vi "Test1_1b_ASIC.vi"(0 "Instrument VISA in":T1={"AWG VISA"="generadorpulsos", "Oscilloscope  VISA "="Oscilloscope", "Integration Board IP"="172.16.7.43", "connection ID"=refnum, "report out"=refnum, "report file path"=path "C:/Documents and Settings/CTA_LAB01/Desktop/L0_Asic/L0 Asic Test Data"}, 1 "threshold":i32[][](array[numeric]), 2 "Serial Number":string, 5 "quantity":i32=3, 7 "Cycles Burst":i32=10000, 11 "error in":errorcluster={"status"=FALSE, "code"=0, "source"="VISA Write in Test2_3a_ASIC_fast.vi->test_sum_ASIC.vi"}, 12 "channel array":i32[](array[numeric])=[0, 1, 2, 3, 4, 5, 6], 13 "Voltages comprobation":dbl[](array[numeric])=[0.05, 0.1, 0.2, 0.5, 0.8, 0.5, 0.6, 0.7, 0.8, 1.0]) -> (4 "Instrument VISA out":T1, 15 "error out":errorcluster)   [LabVIEW 2009]
uses:
  <vilib>/Utility/NIReport.llb/NI_report.lvclass
  <vilib>/Utility/NIReport.llb/HTML/NI_HTML.lvclass
  <instrlib>/Agilent 81150/Agilent 81150.lvlib
  L0_Asic/L0 Asic Test Folder v9/C/Program Files/National Instruments/LabVIEW 2012/instr.lib/Agilent 8000 Series/Agilent 8000 Series.lvlib
panel:
  out "read buffer 4":string="V amptd(f2),1.074E+00,0,1.056E+00,1.087E+00,1.0690E+00,5.5E-03,9.4E+01,+ width(f2),2.90015E-09,0,2.90015E-09,2.95960E-09,2.925838E-09,1.2702E-11,9.4E+01,V amptd(1),5.5E-02,0,4.8E-02,6.7E-02,5.55E-02,3.5E-03,9.4E+01,+ width(f1),9.99999E+37,5,9.99999E+37,9.99999E+37,9.99999E+37,9.99999E+37,9.99999E+37,Time(f1-f2),6.26722E-09,0,6.20145E-09,6.35270E-09,6.264189E-09,3.2805E-11,9.4E+01\n"
  out "report file path":path=path "C:/Documents and Settings/CTA_LAB01/Desktop/L0_Asic/L0 Asic Test Data"
  out "Array":i32[](array[numeric])=[2, 3, 5]
  out "points quantity":dbl=94.0
  out "ouput data array":dbl[](array[numeric])=[0.75, 42.0, 0.0, 63.0, 1.0, 1.069, 0.0055, 2.925838e-09, 1.2702e-11, 0.0555, 0.0035, 9.99999e+37, 9.99999e+37, 6.264189e-09, 3.2805e-11, 94.0]
  out "read buffer 3":string="V amptd(f2),1.074E+00,0,1.056E+00,1.087E+00,1.0690E+00,5.5E-03,9.4E+01,+ width(f2),2.90015E-09,0,2.90015E-09,2.95960E-09,2.925838E-09,1.2702E-11,9.4E+01,V amptd(1),5.5E-02,0,4.8E-02,6.7E-02,5.55E-02,3.5E-03,9.4E+01,+ width(f1),9.99999E+37,5,9.99999E+37,9.99999E+37,9.99999E+37,9.99999E+37,9.99999E+37,Time(f1-f2),6.26722E-09,0,6.20145E-09,6.35270E-09,6.264189E-09,3.2805E-11,9.4E+01\n"
  in  "Voltage":dbl[](array[numeric])=[0.05, 0.1, 0.2, 0.5, 0.8]
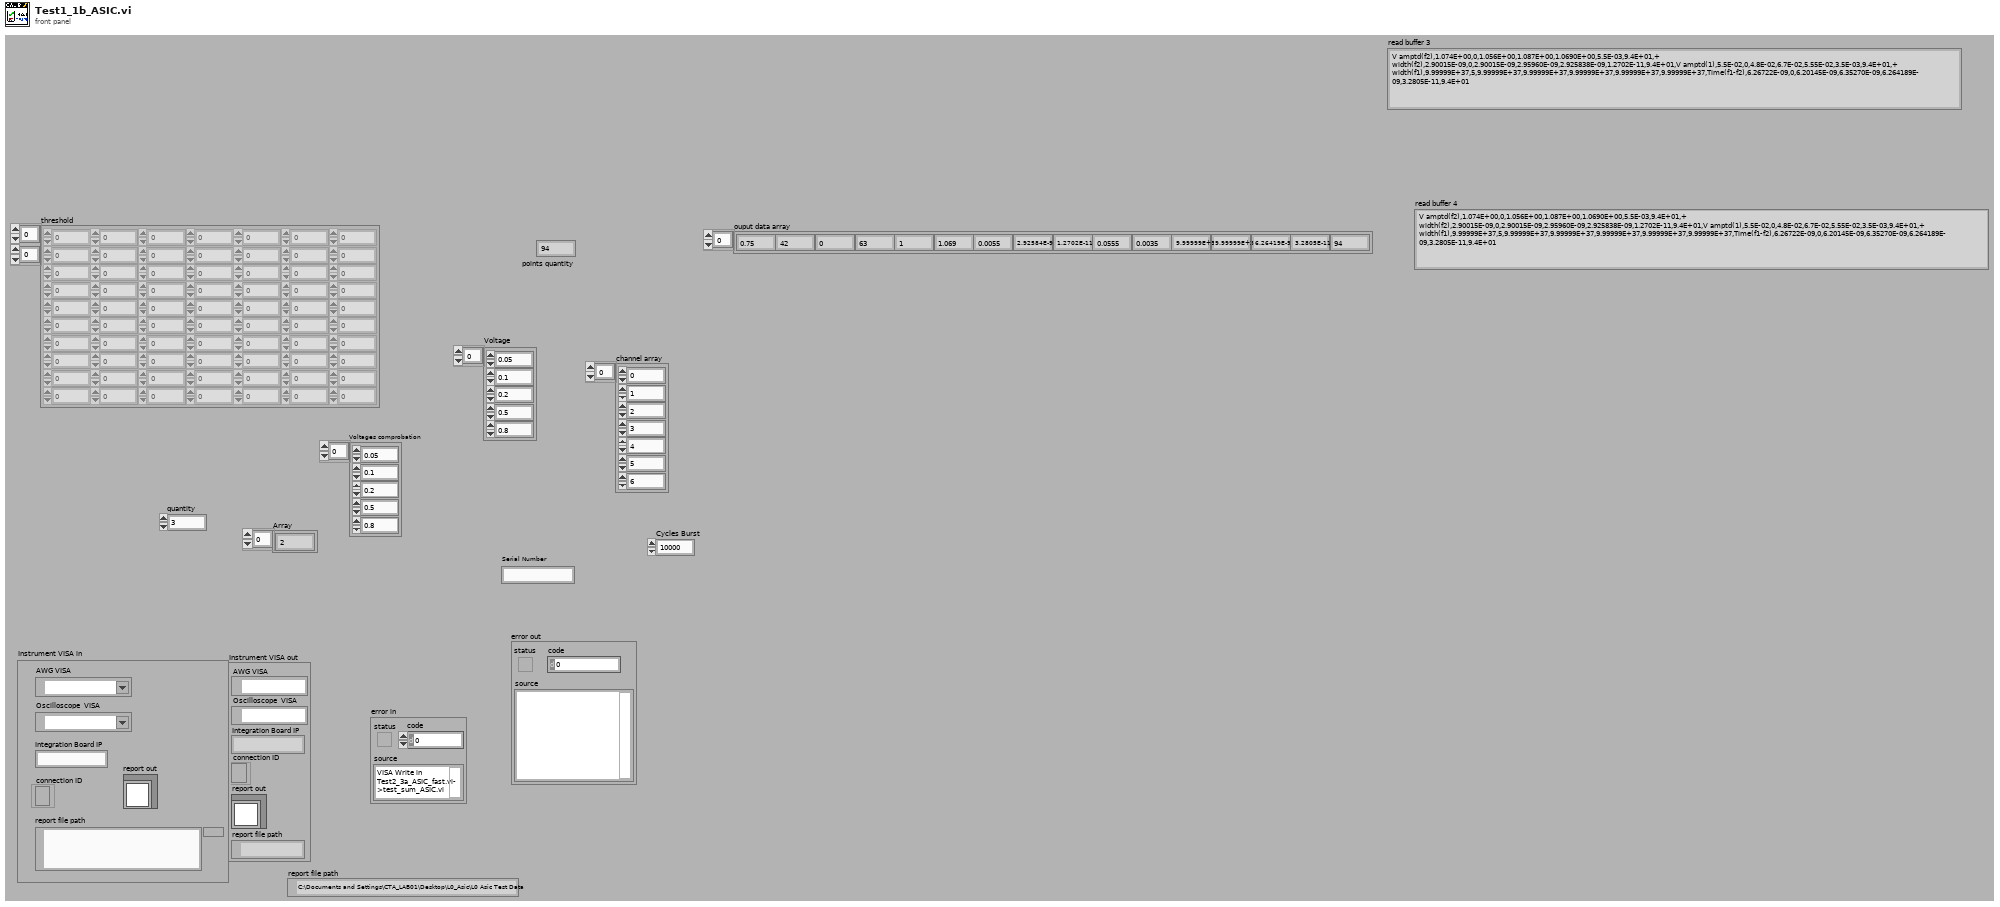
[diagram p1: front panel]
types:
  T1 = cluster{"AWG VISA":refnum<visa-resource-name>, "Oscilloscope  VISA ":refnum<visa-resource-name>, "Integration Board IP":string, "connection ID":refnum<k5>, "report out":refnum<class "NI_report.lvclass">, "report file path":path}
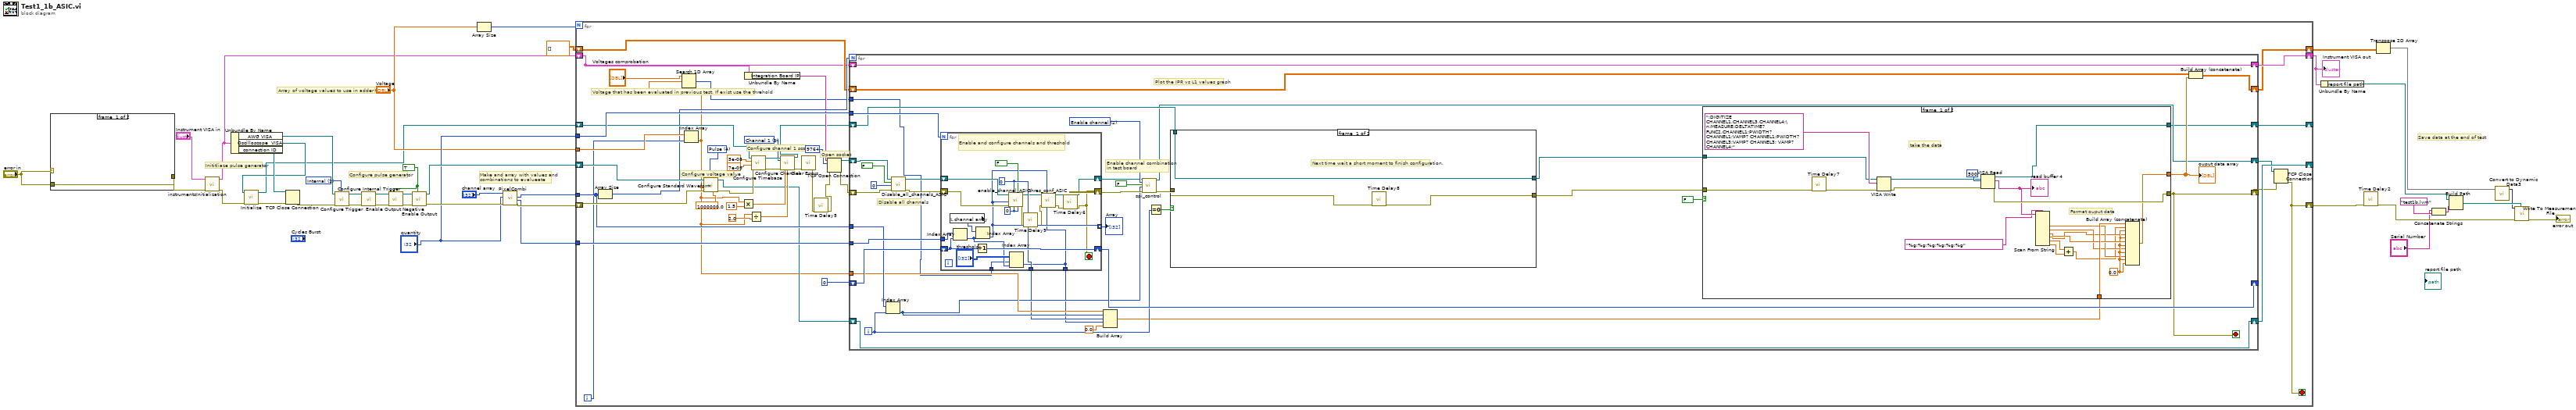
[diagram p0: block diagram]
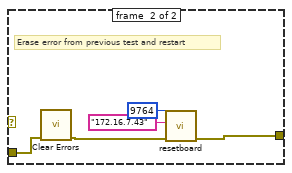
[diagram p2: hidden frame]
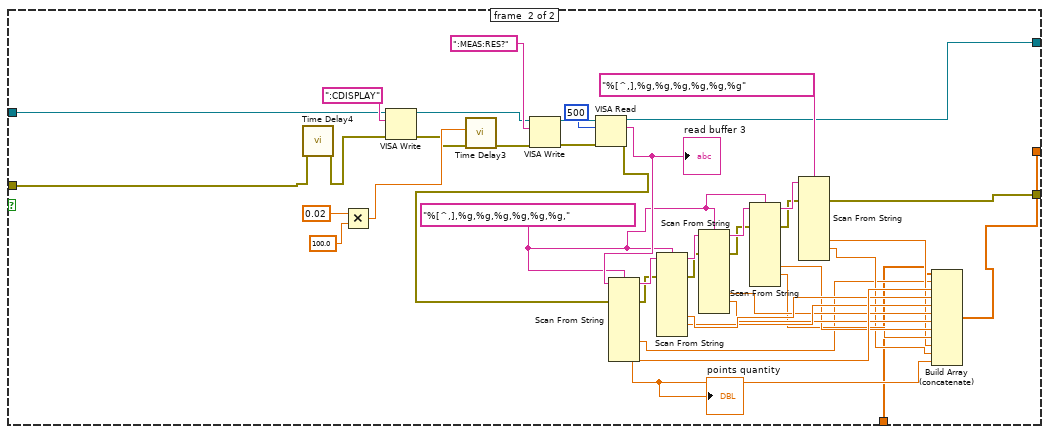
[diagram p3: hidden frame]
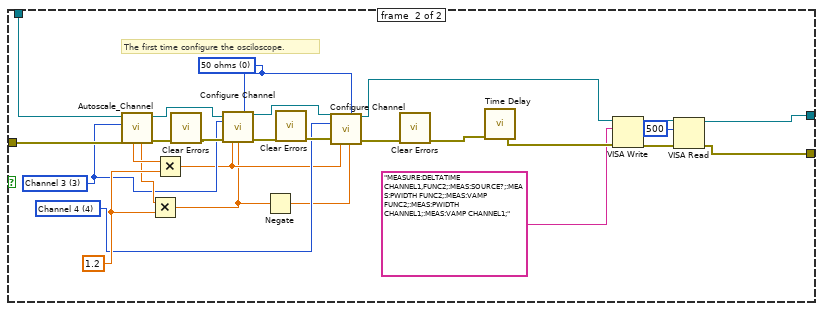
[diagram p4: hidden frame]
diagram:
  w22 = u16 1 items=["Immediate", "Internal", "External", "Software Trigger Function"] ("Trigger Source (0: Immediate)")
  w9 = TRUE ("Enable Output (T: Enable)")
  # "Save data at the end of test"
  # "Array of voltage values to use in adder test"
  # "Make and array with values and \ncombinations to evalueate"
  # "Configure pulse generator"
  # "Inititliaze pulse generator"
  n1 = case shown="No Error" "error in" {
    tunnel: "error in" -> [w42 w44]
    tunnel: [w42 w47] -> w18
    frame #0 {
    }
    frame #1 {
      # "Erase error from previous test and restart"
      n2 = call <vilib>:"Clear Errors.vi"("error in (no error)"=w44) -> ("error out"=w43:errorcluster)  [unwired: 6 in]
      n3 = call "resetboard.vi"("error in (no error)"=w43, "address"="172.16.7.43", "remote port or service name"=u16 9764) -> ("error out"=w47:errorcluster)  [unwired: 7 in, 1 out]
    }
  }
  n4 = call "instrumentsInitialization.vi"("error in"=w18, "Instrument VISA in"="Instrument VISA in") -> ("error out"=w7:errorcluster, "Instrument VISA out"=w15:T1)  [unwired: 8 in]
  n5 = Unbundle By Name(w15) -> ("AWG VISA"=w25:refnum<visa-resource-name>, "Oscilloscope  VISA"=w5:refnum<visa-resource-name>, "connection ID"=w17:refnum<k5>)
  n6 = call "Initialize.vi"("error in (no error)"=w7, "VISA resource name"=w5) -> ("error out"=w6:errorcluster, "VISA resource name out"=w4:refnum<visa-resource-name>)  [unwired: 8 in]
  n7 = TCP Close Connection(connection ID=w17, error in (no error)=w6) -> (error out=w16:errorcluster)  [unwired: 1 in, 1 out]
  n8 = call <instrlib>:"Configure Trigger.vi"("Trigger Source (0: Immediate)"=w22, "error in (no error)"=w16, "VISA resource name"=w25) -> ("error out"=w23:errorcluster, "VISA resource name out"=w24:refnum<visa-resource-name>)  [unwired: 7 in]
  n9 = call <instrlib>:"Configure Internal Trigger.vi"("error in (no error)"=w23, "VISA resource name"=w24) -> ("error out"=w11:errorcluster, "VISA resource name out"=w12:refnum<visa-resource-name>)  [unwired: 8 in]
  n10 = call <instrlib>:"Enable Output Negative.vi"("Enable Output (T: Enable)"=w9, "error in (no error)"=w11, "VISA resource name"=w12) -> ("error out"=w10:errorcluster, "VISA resource name out"=w13:refnum<visa-resource-name>)  [unwired: 7 in]
  n11 = call <instrlib>:"Enable Output.vi"("Enable Output (T: Enable)"=w9, "error in (no error)"=w10, "VISA resource name"=w13) -> ("error out"=w41:errorcluster, "VISA resource name out"=w39:refnum<visa-resource-name>)  [unwired: 7 in]
  n12 = Array Size(array="Voltage") -> (size(s)=w32:i32)
  n13 = call "PixelCombi.vi"("error in"=w41, "quantity"="quantity", "array"="channel array") -> ("error out"=w40:errorcluster, "Channels"=w38:i32[], "Combination Array"=w37:i16[])  [unwired: 6 in]
  n14 = for {
    N: w32 -> [_]
    tunnel: w38 -> [w88]
    tunnel: w37 -> [w87]
    shift-right: [w76] -> w26
    shift-left: w40 -> [w90]
    tunnel: "Voltage" -> [w86]
    tunnel: "quantity" -> [w84]
    shift-right: [w80] -> w14
    shift-left: w15 -> [w51]
    shift-right: [w79] -> w8
    shift-left: dbl[][] [] -> [w81]
    shift-right: [w77] -> _
    shift-left: w39 -> [w89]
    shift-right: [w78] -> _
    shift-left: w4 -> [w83]
    i -> [w85]
    stop <- w76 stop-if-true
    w66 = 1 items=["Channel 1"=1, "Channel 2"=2, "Channel 3"=3, "Channel 4"=4] ("Channel (1: Channel 1)")
    w75 = u16 4 items=["Sine", "Square", "Ramp Up", "Ramp Down", "Pulse", "Noise", "DC"] ("Waveform (0: Sine)")
    # "Open socket"
    # "Configure channel 1 scope"
    # "Configure voltage value"
    # "Voltage that has been evaluated in previous test. If exist use the threhold"
    n15 = Array Size(array=w87) -> (size(s)=w82:i32)
    n16 = Index Array(array=w86, index=w85) -> (element=w50:dbl)
    n17 = Search 1D Array(1D array="Voltages comprobation", element=w50) -> (index of element=w48:i32)  [unwired: 1 in]
    n18 = call <instrlib>:"Configure Standard Waveform.vi"("Frequency (1000.0 Hz)"=1000000.0, "Waveform (0: Sine)"=w75, "error in (no error)"=w90, "Amplitude (1.0 Vpp)"=w50, "VISA resource name"=w89) -> ("error out"=w72:errorcluster, "VISA resource name out"=w54:refnum<visa-resource-name>)  [unwired: 5 in]
    n19 = Multiply(x=w50, y=1.5) -> (x*y=w65:dbl)
    n20 = Unbundle By Name(w51) -> ("Integration Board IP"=w62:string)
    n21 = Divide(x=w50, y=2.0) -> (x/y=w59:dbl)
    n22 = call "Configure Timebase.vi"("error in (no error)"=w72, "Position (0.0 s)"=7e-09, "Timebase (0.005 s)"=5e-08, "VISA resource name"=w83) -> ("error out"=w71:errorcluster, "VISA resource name out"=w69:refnum<visa-resource-name>)  [unwired: 6 in]
    n23 = call "Configure Channel.vi"("VISA resource name"=w69, "Channel (1: Channel 1)"=w66, "error in (no error)"=w71, "Vertical Range (2.0 V)"=w65, "Vertical Offset (0.0 V)"=w59) -> ("VISA resource name out"=w58:refnum<visa-resource-name>, "error out"=w70:errorcluster)  [unwired: 9 in]
    n24 = call <vilib>:"Clear Errors.vi"("error in (no error)"=w70) -> ("error out"=w53:errorcluster)  [unwired: 6 in]
    n25 = call "Time Delay5"("error in (no error)"=w53) -> ("error out"=w52:errorcluster)  [unwired: 10 in]
    n26 = TCP Open Connection(address=w62, remote port or service name=u16 9764, error in (no error)=w52) -> (connection ID=w55:refnum<k5>, error out=w63:errorcluster)  [unwired: 2 in]
    n27 = for {
      N: w82 -> [_]
      tunnel: w87 -> [w125]
      tunnel: w88 -> [w126]
      shift-right: [w127] -> _
      shift-left: i16 0 ("element") -> [w128]
      shift-right: [w106] -> w57
      shift-left: w63 -> [w118]
      tunnel: w84 -> [w124]
      shift-right: [w119] -> w79
      shift-left: w81 -> [w120]
      shift-right: [w107] -> w56
      shift-left: w55 -> [w105]
      tunnel: w50 -> [w103]
      shift-right: [w99] -> w78
      shift-left: w58 -> [w112]
      shift-right: [w98] -> w77
      shift-left: w54 -> [w98]
      shift-right: [w93] -> w80
      shift-left: w51 -> [w93]
      tunnel: w48 -> [w91]
      i -> [w110]
      stop <- w106 stop-if-true
      w117 = u16 2 items=["Attenuation", "Clipping", "Enable channel", "Delay line", "ASIC"] ("Device")
      # "Enable channel combination \nin test board"
      # "Disable all channels"
      # "Plot the IPR vs L1 values graph"
      n28 = Index Array(array=w125, index=w110) -> (element=w102:i16)
      n29 = call "Disable_all_channels_ASIC.vi"("error in"=w118, "id_in"=0 ("Data"), "Clip_en_b"=FALSE, "connection ID"=w105) -> ("error out"=w122:errorcluster, "connection ID out"=w121:refnum<k5>)  [unwired: 5 in, 1 out]
      n30 = for {
        N: w124 -> [_]
        shift-right: [w239] -> w127
        shift-left: w128 -> [w240]
        tunnel: w126 -> [w238]
        shift-right: [w227] -> w115
        shift-left: w122 -> [w236]
        shift-right: [w230] -> w114
        shift-left: w121 -> [w235]
        tunnel: [w229] -> w104 mode=indexing
        tunnel: [w234] -> w101
        tunnel: [w228] -> w94
        tunnel: w91 -> [w223]
        stop <- w227 stop-if-true
        w232 = u32 0 ("Ib_clipVb")
        w234 = u32 0 ("Att gain")
        # "Enable and configure channels and threshold"
        n31 = local read "channel array"() -> (w237:i32[])
        n32 = Index Array(array=w238, index=w240) -> (element=w224:i32)
        n33 = Increment(x=w240) -> (x+1=w239:i16)
        n34 = Index Array(array=w237, index=w224) -> (element=w229:i32)
        n35 = call "enable_channel_ASIC.vi"("Clip_sel_b"=w232, "maj/sum"=FALSE, "Ib_clipVb"=w232, "Att gain"=w234, "error in"=w236, "Channel"=w229, "connection ID"=w235) -> ("error out"=w221:errorcluster, "connection ID out"=w231:refnum<k5>)  [unwired: 2 in, 1 out]
        n36 = Index Array(array="threshold", index (row)=w223, index (col)=w224) -> (element=w228:i32)
        n37 = call "Time Delay9"("error in (no error)"=w221) -> ("error out"=w222:errorcluster)  [unwired: 10 in]
        n38 = call "thres_conf_ASIC.vi"("threshold"=w228, "Ring"=w229, "error out 3"=w222, "connection ID"=w231) -> ("error out 2"=w226:errorcluster, "connection ID out"=w230:refnum<k5>)  [unwired: 4 in, 2 out]
        n39 = call "Time Delay6"("error in (no error)"=w226) -> ("error out"=w227:errorcluster)  [unwired: 10 in]
      }
      "Array" <- w104
      n40 = Build Array(w103, w102, w101, w94, 0.0 ("element")) -> (w100:dbl[])
      n41 = call "spi_control.vi"("connection ID"=w114, "Device"=w117, "Read/#write"=FALSE, "Data"=w102, "error out 3"=w115) -> ("connection ID out"=w107:refnum<k5>, "error out 2"=w113:errorcluster)  [unwired: 7 in, 6 out]
      n42 = Equal To 0?(x=w110) -> (x = 0?=w111:bool)
      n43 = case shown="True" w111 {
        tunnel: [w191 w200] -> w96
        tunnel: w113 -> [w192 w206]
        tunnel: w112 -> [w193 w207]
        tunnel: [w193 w209] -> w109
        frame #0 {
          # "Next time wait a short moment to finish configuration."
          n44 = call "Time Delay8"("error in (no error)"=w192) -> ("error out"=w191:errorcluster)  [unwired: 10 in]
        }
        frame #1 {
          w210 = u32 0 items=["50 ohms", "1 Mohms"] ("Input Impedance (1: 1 Mohms)")
          w198 = 3 items=["Channel 1"=1, "Channel 2"=2, "Channel 3"=3, "Channel 4"=4] ("Channel (1: Channel 1)")
          w197 = 4 items=["Channel 1"=1, "Channel 2"=2, "Channel 3"=3, "Channel 4"=4] ("Channel (1: Channel 1)")
          w203 = 1.2 ("y")
          # "The first time configure the osciloscope."
          n45 = call "Autoscale_Channel.vi"("error in"=w206, "Channel"=w198, "VISA resource name"=w207) -> ("error out"=w217:errorcluster, "VISA resource name out"=w220:refnum<visa-resource-name>, "Offset"=w199:dbl, "VerticalRange"=w214:dbl)  [unwired: 5 in]
          n46 = Multiply(x=w199, y=w203) -> (x*y=w195:dbl)
          n47 = Multiply(x=w214, y=w203) -> (x*y=w196:dbl)
          n48 = call <vilib>:"Clear Errors.vi"("error in (no error)"=w217) -> ("error out"=w218:errorcluster)  [unwired: 6 in]
          n49 = call "Configure Channel.vi"("VISA resource name"=w220, "Input Impedance (1: 1 Mohms)"=w210, "Channel (1: Channel 1)"=w198, "error in (no error)"=w218, "Vertical Range (2.0 V)"=w196, "Vertical Offset (0.0 V)"=w195) -> ("VISA resource name out"=w215:refnum<visa-resource-name>, "error out"=w219:errorcluster)  [unwired: 8 in]
          n50 = Negate(x=w195) -> (-x=w194:dbl)
          n51 = call <vilib>:"Clear Errors.vi"("error in (no error)"=w219) -> ("error out"=w208:errorcluster)  [unwired: 6 in]
          n52 = call "Configure Channel.vi"("VISA resource name"=w215, "Input Impedance (1: 1 Mohms)"=w210, "Channel (1: Channel 1)"=w197, "error in (no error)"=w208, "Vertical Range (2.0 V)"=w196, "Vertical Offset (0.0 V)"=w194) -> ("VISA resource name out"=w204:refnum<visa-resource-name>, "error out"=w216:errorcluster)  [unwired: 8 in]
          n53 = call <vilib>:"Clear Errors.vi"("error in (no error)"=w216) -> ("error out"=w205:errorcluster)  [unwired: 6 in]
          n54 = call "Time Delay"("error in (no error)"=w205) -> ("error out"=w202:errorcluster)  [unwired: 10 in]
          n55 = VISA Write(VISA resource name=w204, write buffer="MEASURE:DELTATIME CHANNEL1,FUNC2;:MEAS:SOURCE?;:MEAS:PWIDTH FUNC2;:MEAS:VAMP FUNC2;:MEAS:PWIDTH CHANNEL1;:MEAS:VAMP CHANNEL1;", error in (no error)=w202) -> (VISA resource name out=w213:refnum<visa-resource-name>, error out=w212:errorcluster)  [unwired: 1 out]
          n56 = VISA Read(VISA resource name=w213, byte count=u32 500, error in (no error)=w212) -> (VISA resource name out=w209:refnum<visa-resource-name>, error out=w200:errorcluster)  [unwired: 2 out]
        }
      }
      n57 = case shown="False" FALSE {
        tunnel: w109 -> [w146 w158]
        tunnel: [w141 w156] -> w108
        tunnel: [w144 w155] -> w106
        tunnel: w100 -> [w142 w153]
        tunnel: [w143 w152] -> w99
        tunnel: w96 -> [w145 w150]
        frame #0 {
          w137 = 0.0 ("output 7")
          # "Format ouput data"
          # "take the data"
          n58 = call "Time Delay7"("error in (no error)"=w145) -> ("error out"=w147:errorcluster)  [unwired: 10 in]
          n59 = VISA Write(VISA resource name=w146, write buffer=":DIGITIZE CHANNEL1,CHANNEL3,CHANNEL4;\n:MEASURE:DELTATIME? FUNC2,CHANNEL1;PWIDTH? CHANNEL1;VAMP? CHANNEL1;PWIDTH? CHANNEL3;VAMP? CHANNEL3; VAMP? CHANNEL4;", error in (no error)=w147) -> (VISA resource name out=w140:refnum<visa-resource-name>, error out=w139:errorcluster)  [unwired: 1 out]
          n60 = VISA Read(VISA resource name=w140, byte count=u32 500, error in (no error)=w139) -> (VISA resource name out=w143:refnum<visa-resource-name>, read buffer=w136:string, error out=w144:errorcluster)  [unwired: 1 out]
          "read buffer 4" <- w136
          n61 = Scan From String(format string="%g;%g;%g;%g;%g;%g", input string=w136) -> (output 1=w134:dbl, output 2=w133:dbl, output 3=w138:dbl, output 4=w132:dbl, output 5=w131:dbl, output 6=w130:dbl)  [unwired: 8 in, 3 out]
          n62 = Add(x=w131, y=w130) -> (x+y=w129:dbl)
          n63 = Build Array (concatenate)(w142, w129, w137, w132, w137, w138, w137, w133, w137, w134, w137, w137) -> (w141:dbl[])
        }
        frame #1 {
          w176 = "%[^,],%g,%g,%g,%g,%g,%g," ("format string")
          n64 = call "Time Delay4"("error in (no error)"=w150) -> ("error out"=w151:errorcluster)  [unwired: 10 in]
          n65 = Multiply(x=0.02, y=100.0) -> (x*y=w183:dbl)
          n66 = VISA Write(VISA resource name=w158, write buffer=":CDISPLAY", error in (no error)=w151) -> (VISA resource name out=w161:refnum<visa-resource-name>, error out=w159:errorcluster)  [unwired: 1 out]
          n67 = call "Time Delay3"("error in (no error)"=w159, "Delay Time (s)"=w183) -> ("error out"=w182:errorcluster)  [unwired: 9 in]
          n68 = VISA Write(VISA resource name=w161, write buffer=":MEAS:RES?", error in (no error)=w182) -> (VISA resource name out=w190:refnum<visa-resource-name>, error out=w189:errorcluster)  [unwired: 1 out]
          n69 = VISA Read(VISA resource name=w190, byte count=u32 500, error in (no error)=w189) -> (VISA resource name out=w152:refnum<visa-resource-name>, read buffer=w186:string, error out=w166:errorcluster)  [unwired: 1 out]
          "read buffer 3" <- w186
          n70 = Scan From String(format string=w176, input string=w186, error in=w166) -> (remaining string=w180:string, error out=w162:errorcluster, output 5=w154:dbl, output 6=w181:dbl, output 7=w167:dbl)  [unwired: 12 in, 1 out]
          "points quantity" <- w167
          n71 = Scan From String(format string=w176, input string=w180, error in=w162) -> (remaining string=w177:string, error out=w163:errorcluster, output 5=w174:dbl, output 6=w173:dbl)  [unwired: 13 in, 1 out]
          n72 = Scan From String(format string=w176, input string=w177, error in=w163) -> (remaining string=w178:string, error out=w164:errorcluster, output 5=w172:dbl, output 6=w171:dbl)  [unwired: 13 in, 1 out]
          n73 = Scan From String(format string=w176, input string=w178, error in=w164) -> (remaining string=w179:string, error out=w165:errorcluster, output 5=w170:dbl, output 6=w169:dbl)  [unwired: 13 in, 1 out]
          n74 = Scan From String(format string="%[^,],%g,%g,%g,%g,%g,%g", input string=w179, error in=w165) -> (error out=w155:errorcluster, output 5=w157:dbl, output 6=w168:dbl)  [unwired: 13 in, 2 out]
          n75 = Build Array (concatenate)(w153, w154, w181, w174, w173, w172, w171, w170, w169, w157, w168, w167) -> (w156:dbl[])
        }
      }
      "ouput data array" <- w108
      n76 = Build Array (concatenate)(w120, w108) -> (w119:dbl[][])
    }
    n77 = TCP Close Connection(connection ID=w56, error in (no error)=w57) -> (error out=w76:errorcluster)  [unwired: 1 in, 1 out]
  }
  "Instrument VISA out" <- w14
  n78 = Unbundle By Name(w14) -> ("report file path"=w35:path)
  n79 = call "Time Delay2"("error in (no error)"=w26) -> ("error out"=w33:errorcluster)  [unwired: 10 in]
  n80 = Transpose 2D Array(2D array=w8) -> (transposed array=w20:dbl[][])
  n81 = Concatenate Strings("Serial Number", "test1b.lvm" ("string")) -> (w3:string)
  n82 = Build Path(base path=w35, name or relative path=w3) -> (appended path=w34:path)
  n83 = call "Convert to Dynamic Data3"("2D Array"=w20) -> ("Dynamic Data Type"=w21:dynamicdata)  [unwired: 3 in]
  n84 = call "Write To Measurement File"("Signals"=w21, "error in (no error)"=w33, "Filename"=w34) -> ("error out"=→"error out":errorcluster)  [unwired: 14 in, 2 out]
